vi "serpenbot_DDPG_learing_parallel_old_camera_2.vi"() -> ()   [LabVIEW 2020]
uses:
  <vilib>/Analysis/Matrix/Datatypes/RealMatrix.ctl
  <vilib>/Analysis/Matrix/NI_Matrix.lvlib
  <vilib>/Analysis/NI_AALBase.lvlib
  <vilib>/Analysis/baseanly.llb/Real A x B.vi
  <vilib>/Analysis/NI_AALPro.lvlib
  <vilib>/Analysis/Matrix/Numeric/Subtract/Subtract - RM,RM.vi
  <vilib>/Analysis/_algsub.llb/Real PseudoInverse Matrix.vi
panel:
  out "camera_value 2":T1
  out "appended array 3":T1
  out "error out Y":errorcluster
  out "error out X":errorcluster
  out "laser control value":dbl[](array[numeric])
  out "current y":dbl
  out "current x":dbl
  out "control_loop_time":u32
  in  "stop":bool
  in  "Logging":bool caption="Enable"
  in  "k":T1
  in  "Diode Current\nSetting":dbl=3.0
  in  "Laser Repetition\nFrequency":i32=50000
  in  "VISA resource name":refnum<visa-resource-name>="COM14"
  in  "baud rate (9600)":u32=9600
  out "error out":errorcluster
  out "Identification system 1":string
  out "Conn. axes system 1":string[](array[string])
  out "Identification system 2":string
  out "Conn. axes system  2":string[](array[string])
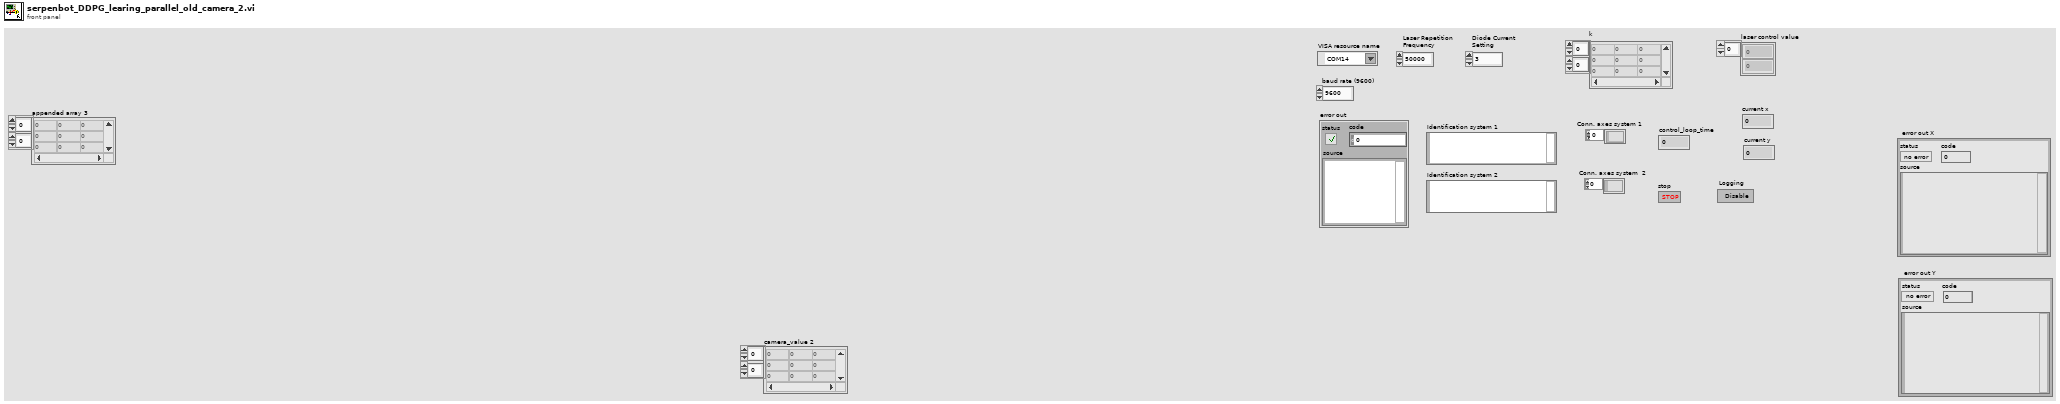
[diagram p1: front panel]
types:
  T1 = typedef "NI_Matrix.lvlib/RealMatrix.ctl" = dbl[][]
  T2 = cluster{"RS232 settings":cluster{"Portnumber":i32, "Baudrate":u16}, "USB settings":cluster{"S/N":string, "USB Search?":bool}, "TCP/IP settings":cluster{"Host address/name":string, "Port":i32, "Board":i32, "TCP/IP Search?":bool}}
  T3 = cluster{"Check FRF?":bool, "Referencing mode":enum16{"FRF (-> FNL)", "FRF", "FNL", "FPL", "RON OFF"}[]}
  T4 = cluster{"Force?":bool, "Dialog?":bool, "Stages":string[]}
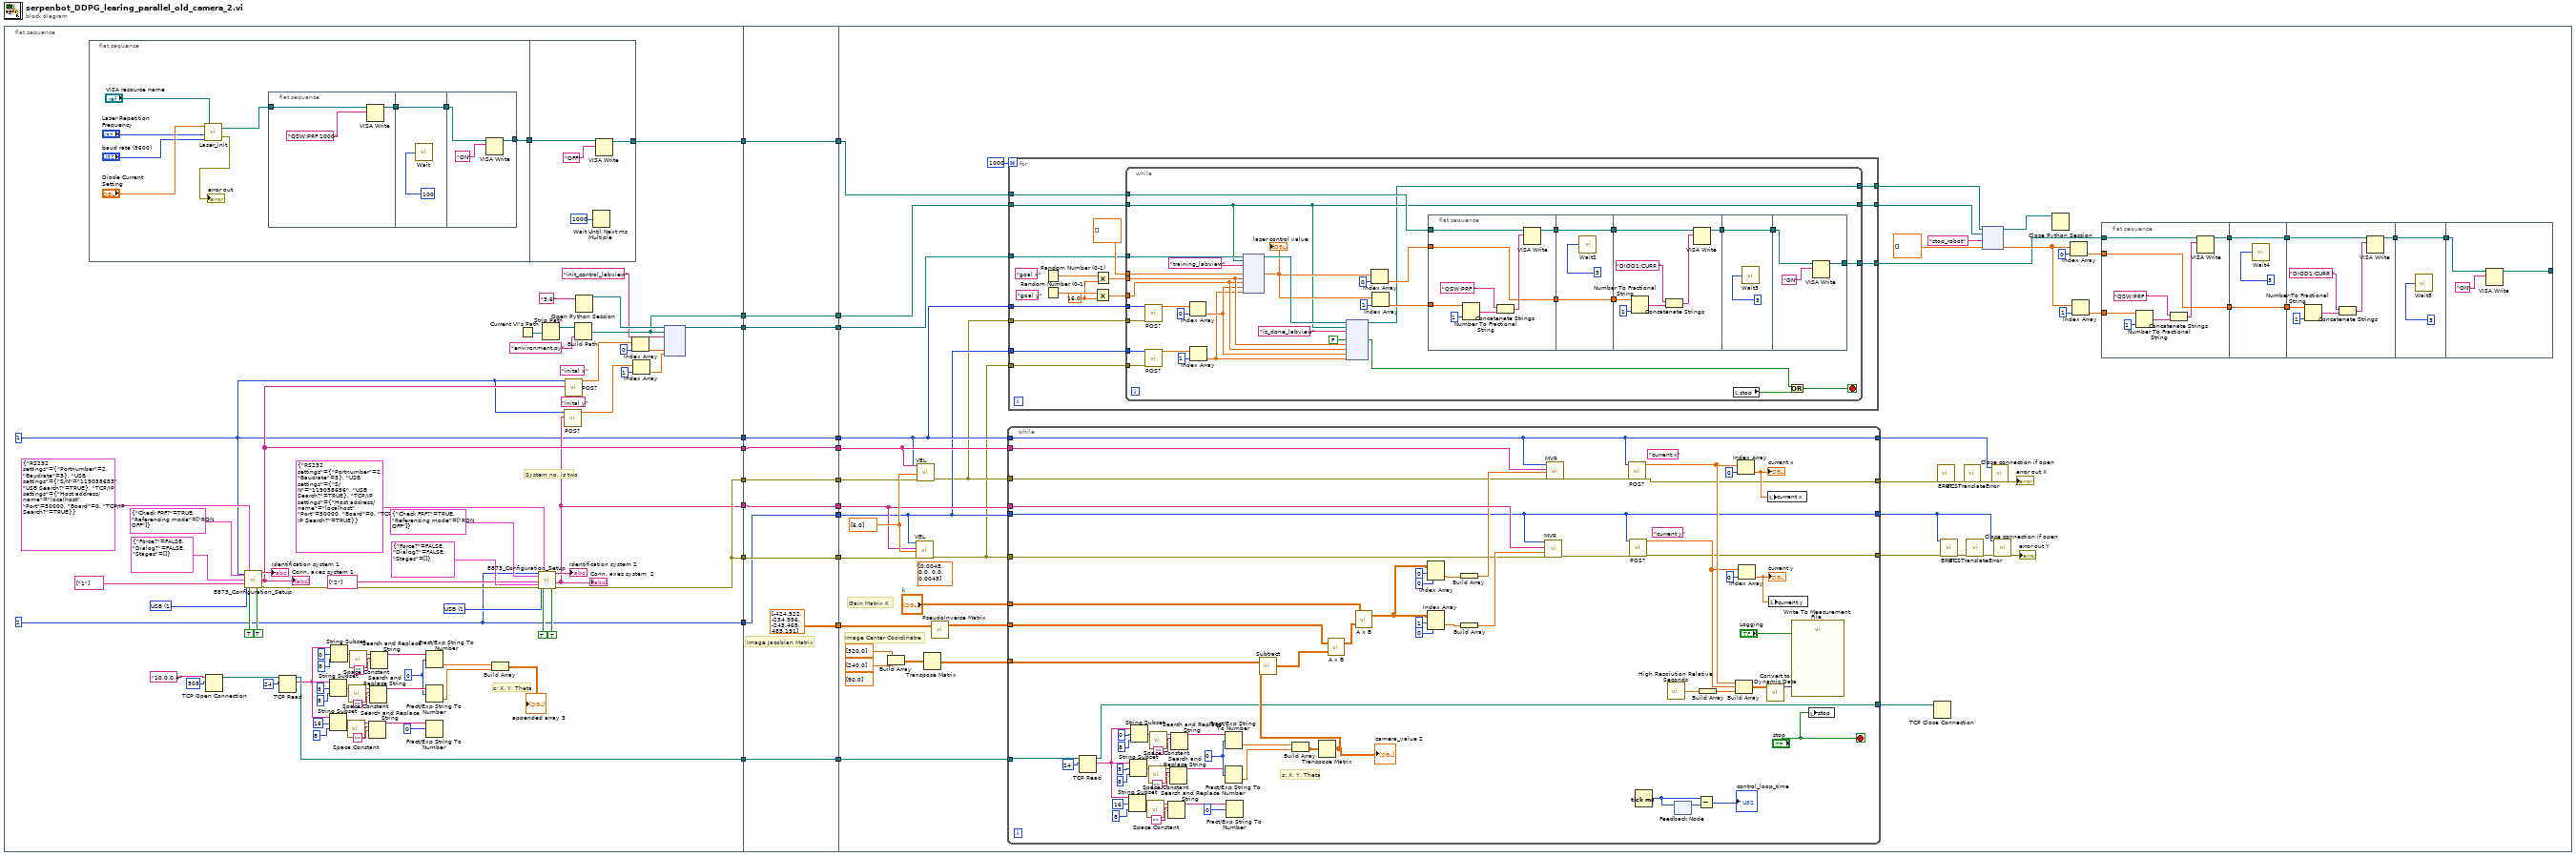
[diagram p0: block diagram]
diagram:
  n1 = flat-sequence {
    tunnel: [w87] -> w21
    tunnel: [w57] -> w20
    tunnel: [w59] -> w19
    tunnel: [w68] -> w18
    tunnel: [w58] -> w17
    tunnel: [w69] -> w16
    tunnel: [w68] -> w15
    tunnel: [w61] -> w14
    tunnel: [w60] -> w13
    tunnel: [w22] -> w2
    tunnel: w21 -> [w120]
    tunnel: [w120] -> w12
    tunnel: w20 -> [w119]
    tunnel: w19 -> [w118]
    tunnel: w18 -> [w117]
    tunnel: w17 -> [w116]
    tunnel: w16 -> [w114]
    tunnel: [w119] -> w11
    tunnel: [w118] -> w10
    tunnel: [w117] -> w9
    tunnel: [w116] -> w8
    tunnel: w15 -> [w115]
    tunnel: [w115] -> w7
    tunnel: [w114] -> w6
    tunnel: [T1 [[-424.522, -234.956], [-243.465, 485.191]] ("J_init 2")] -> w5
    tunnel: w14 -> [w112]
    tunnel: w13 -> [w111]
    tunnel: [w112] -> w4
    tunnel: [w111] -> w3
    tunnel: w2 -> [w110]
    tunnel: [w110] -> w1
    tunnel: w12 -> [w141]
    tunnel: w11 -> [w125]
    tunnel: w10 -> [w162]
    tunnel: w9 -> [w165]
    tunnel: w8 -> [w161]
    tunnel: w7 -> [w164]
    tunnel: w6 -> [w124]
    tunnel: w5 -> [w163]
    tunnel: w4 -> [w143]
    tunnel: w3 -> [w142]
    tunnel: w1 -> [w127]
    frame #0 {
      w36 = 0
      (unwired) "inital y"
      (unwired) "inital x"
      w72 = u16 1 items=["RS232", "USB", "TCP/IP"] ("Interface")
      w75 = u16 1 items=["RS232", "USB", "TCP/IP"] ("Interface")
      w69 = 2 ("System no.")
      w57 = 1 ("System no.")
      # "s: X, Y, Theta"
      # "System no. is two"
      n2 = flat-sequence {
        tunnel: [w89] -> w88
        tunnel: w88 -> [w107]
        tunnel: [w106] -> w87
        frame #0 {
          n3 = call "Laser_init.vi"("baud rate (9600)"="baud rate (9600)", "Laser Repetition\nFrequency"="Laser Repetition\nFrequency", "VISA resource name"="VISA resource name", "Diode Current\nSetting"="Diode Current\nSetting") -> ("error out"=→"error out":errorcluster, "VISA Refnum out"=w90:refnum<visa-resource-name>)
          n4 = flat-sequence {
            tunnel: w90 -> [w100]
            tunnel: [w99] -> w97
            tunnel: w97 -> [w102]
            tunnel: [w102] -> w96
            tunnel: w96 -> [w103]
            tunnel: [w104] -> w89
            frame #0 {
              n5 = VISA Write(VISA resource name=w100, write buffer="QSW:PRF 1000" ("string")) -> (VISA resource name out=w99:refnum<visa-resource-name>)  [unwired: 1 in, 2 out]
            }
            frame #1 {
              n6 = call "Wait"("Count(mSec)"=u32 100) -> ()  [unwired: 1 out]
            }
            frame #2 {
              n7 = VISA Write(VISA resource name=w103, write buffer="ON") -> (VISA resource name out=w104:refnum<visa-resource-name>)  [unwired: 1 in, 2 out]
            }
          }
        }
        frame #1 {
          n8 = Wait Until Next ms Multiple(millisecond multiple=u32 1000) -> ()  [unwired: 1 out]
          n9 = VISA Write(VISA resource name=w107, write buffer="OFF") -> (VISA resource name out=w106:refnum<visa-resource-name>)  [unwired: 1 in, 2 out]
        }
      }
      n10 = TCP Open Connection(address="10.0.0.4", remote port or service name=u16 503) -> (connection ID=w46:refnum<k5>)  [unwired: 3 in, 1 out]
      n11 = call "E873_Configuration_Setup.vi"("System no."=w57, "Referencing"=T3 {"Check FRF?"=TRUE, "Referencing mode"=[enum."RON OFF"]}, "Interface"=w75, "All axes?"=TRUE, "Axes to move"=string[] ["1"], "Interface settings"=T2 {"RS232 settings"={"Portnumber"=2, "Baudrate"=5}, "USB settings"={"S/N"="119058653", "USB Search?"=TRUE}, "TCP/IP settings"={"Host address/name"="localhost", "Port"=50000, "Board"=0, "TCP/IP Search?"=TRUE}}, "Stage selection"=T4 {"Force?"=FALSE, "Dialog?"=FALSE, "Stages"=[]}, "Switch servo on?"=TRUE ("Use dialog to define\nconnected stages?")) -> ("Identification"=→"Identification system 1":string, "Conn. \nAxes"=w59:string[], "error out"=w84:errorcluster)  [unwired: 4 in, 5 out]
      "Conn. axes system 1" <- w59
      n12 = TCP Read(connection ID=w46, bytes to read=24) -> (connection ID out=w22:refnum<k5>, data out=w45:string)  [unwired: 3 in, 1 out]
      n13 = String Subset(string=w45, offset (0)=16, length (rest)=8 ("length (rest)")) -> (substring=w43:string)
      n14 = String Subset(string=w45, offset (0)=8, length (rest)=8 ("length (rest)")) -> (substring=w44:string)
      n15 = String Subset(string=w45, offset (0)=0, length (rest)=8 ("length (rest)")) -> (substring=w42:string)
      n16 = call <vilib>:"Space Constant.vi"() -> ("String"=w41:string)
      n17 = call <vilib>:"Space Constant.vi"() -> ("String"=w40:string)
      n18 = call <vilib>:"Space Constant.vi"() -> ("String"=w39:string)
      n19 = Search and Replace String(input string=w43, search string=w41, replace string="") -> (result string=w47:string)  [unwired: 5 in, 3 out]
      n20 = Search and Replace String(input string=w44, search string=w40, replace string="") -> (result string=w48:string)  [unwired: 5 in, 3 out]
      n21 = Search and Replace String(input string=w42, search string=w39, replace string="") -> (result string=w49:string)  [unwired: 5 in, 3 out]
      n22 = Fract/Exp String To Number(string=w49, offset=w36) -> (number=w37:dbl)  [unwired: 2 in, 1 out]
      n23 = Fract/Exp String To Number(string=w48, offset=w36) -> (number=w38:dbl)  [unwired: 2 in, 1 out]
      n24 = Fract/Exp String To Number(string=w47, offset=0) -> ()  [unwired: 2 in, 2 out]
      n25 = Build Array(w37, w38) -> (→"appended array 3":T1)
      n26 = Current VI's Path() -> (path=w67:path)
      n27 = call "E873_Configuration_Setup.vi"("System no."=w69, "Referencing"=T3 {"Check FRF?"=TRUE, "Referencing mode"=[enum."RON OFF"]}, "Interface"=w72, "All axes?"=TRUE, "Axes to move"=string[] ["2"], "error in"=w84, "Interface settings"=T2 {"RS232 settings"={"Portnumber"=2, "Baudrate"=5}, "USB settings"={"S/N"="119058656", "USB Search?"=TRUE}, "TCP/IP settings"={"Host address/name"="localhost", "Port"=50000, "Board"=0, "TCP/IP Search?"=TRUE}}, "Stage selection"=T4 {"Force?"=FALSE, "Dialog?"=FALSE, "Stages"=[]}, "Switch servo on?"=TRUE ("Use dialog to define\nconnected stages?")) -> ("Identification"=→"Identification system 2":string, "Conn. \nAxes"=w58:string[], "error out"=w68:errorcluster)  [unwired: 3 in, 5 out]
      "Conn. axes system  2" <- w58
      n28 = Strip Path(path=w67) -> (stripped path=w66:path)  [unwired: 1 out]
      n29 = call "POS?.vi"("System no."=w57, "Axes to query"=w58) -> ("Position"=w51:dbl[])  [unwired: 3 in, 14 out]
      n30 = call "POS?.vi"("System no."=w57, "Axes to query"=w59) -> ("Position"=w54:dbl[])  [unwired: 3 in, 14 out]
      n31 = Build Path(base path=w66, name or relative path="environment.py") -> (appended path=w61:path)
      n32 = Open Python Session(python version="3.6" ("Python version")) -> (session out=w63:refnum<k35>)  [unwired: 2 in, 1 out]
      n33 = Index Array(array=w54, index=0) -> (element=w55:dbl)
      n34 = Index Array(array=w51, index=1) -> (element=w52:dbl)
      n35 = node(w63, w61, "init_control_labview" ("function name"), w55, w52) -> (w60:refnum<k35>)  [unwired: 5 in, 3 out]
    }
    frame #1 {
      # "Image Jacobian Matrix"
    }
    frame #2 {
      w166 = dbl[] [6.0] ("Velocity values")
      (unwired) T1 [[0.0045, 0.0], [0.0, 0.0045]] ("J_init 2")
      (unwired) dbl[] [90.0] ("element")
      # "Gain Matrix K"
      # "Image Center Coordinatre"
      n36 = Build Array(dbl[] [320.0] ("element"), dbl[] [240.0] ("element")) -> (w167:T1)
      n37 = call "VEL.vi"("System no."=w124, "Axes to set"=w161, "Velocity values"=w166, "error in"=w164) -> ("error out"=w122:errorcluster)  [unwired: 2 in, 13 out]
      n38 = call "VEL.vi"("System no."=w125, "Axes to set"=w162, "Velocity values"=w166, "error in"=w165) -> ("error out"=w123:errorcluster)  [unwired: 2 in, 13 out]
      n39 = Transpose Matrix(1:w167) -> (0:w158:T1)
      n40 = call-poly <vilib>:"PseudoInverse Matrix.vi"("Input Matrix"=w163) -> ("PseudoInverse Matrix"=w159:T1)  [unwired: 1 in, 1 out]
      n41 = while {
        tunnel: w122 -> [w293]
        tunnel: w124 -> [w274]
        tunnel: w161 -> [w311]
        tunnel: w123 -> [w294]
        tunnel: w162 -> [w310]
        tunnel: w125 -> [w276]
        tunnel: w159 -> [w299]
        tunnel: "k" -> [w298]
        tunnel: w158 -> [w297]
        tunnel: [w276] -> w130
        tunnel: [w275] -> w121
        tunnel: [w274] -> w129
        tunnel: [w273] -> w128
        tunnel: w127 -> [w246]
        tunnel: [w245] -> w126
        stop <- "stop" stop-if-true
        w272 = 0
        (unwired) "current y"
        (unwired) "current x"
        # "s: X, Y, Theta"
        n42 = TCP Read(connection ID=w246, bytes to read=24) -> (connection ID out=w245:refnum<k5>, data out=w253:string)  [unwired: 3 in, 1 out]
        n43 = String Subset(string=w253, offset (0)=16, length (rest)=8 ("length (rest)")) -> (substring=w255:string)
        n44 = String Subset(string=w253, offset (0)=8, length (rest)=8 ("length (rest)")) -> (substring=w254:string)
        n45 = String Subset(string=w253, offset (0)=0, length (rest)=8 ("length (rest)")) -> (substring=w260:string)
        n46 = call <vilib>:"Space Constant.vi"() -> ("String"=w263:string)
        n47 = call <vilib>:"Space Constant.vi"() -> ("String"=w265:string)
        n48 = call <vilib>:"Space Constant.vi"() -> ("String"=w267:string)
        n49 = Search and Replace String(input string=w255, search string=w263, replace string="") -> (result string=w251:string)  [unwired: 5 in, 3 out]
        n50 = Search and Replace String(input string=w254, search string=w265, replace string="") -> (result string=w250:string)  [unwired: 5 in, 3 out]
        n51 = Search and Replace String(input string=w260, search string=w267, replace string="") -> (result string=w249:string)  [unwired: 5 in, 3 out]
        n52 = Fract/Exp String To Number(string=w249, offset=w272) -> (number=w271:dbl)  [unwired: 2 in, 1 out]
        n53 = Fract/Exp String To Number(string=w250, offset=w272) -> (number=w270:dbl)  [unwired: 2 in, 1 out]
        n54 = Fract/Exp String To Number(string=w251, offset=0) -> ()  [unwired: 2 in, 2 out]
        n55 = Build Array(w271, w270) -> (w248:T1)
        n56 = Transpose Matrix(1:w248) -> (0:w247:T1)
        "camera_value 2" <- w247
        n57 = call-poly <vilib>:"Subtract.vi"("Real Matrix B"=w247, "Real Matrix A"=w297) -> ("A - B"=w305:T1)
        n58 = call-poly <vilib>:"A x B.vi"("B"=w305, "A"=w299) -> ("A x B"=w303:T1)  [unwired: 1 out]
        n59 = call-poly <vilib>:"A x B.vi"("B"=w303, "A"=w298) -> ("A x B"=w304:T1)  [unwired: 1 out]
        n60 = Index Array(array=w304, index (row)=0, index (col)=0) -> (element=w296:dbl)
        n61 = Index Array(array=w304, index (row)=1, index (col)=0) -> (element=w295:dbl)
        n62 = Build Array(w296) -> (w302:dbl[])
        n63 = Build Array(w295) -> (w301:dbl[])
        n64 = call "MVR.vi"("System no."=w274, "Axes to move"=w311, "Position values"=w301, "error in"=w293) -> ("error out"=w285:errorcluster)  [unwired: 1 in, 14 out]
        n65 = call "MVR.vi"("System no."=w276, "Axes to move"=w310, "Position values"=w302, "error in"=w294) -> ("error out"=w286:errorcluster)  [unwired: 1 in, 14 out]
        n66 = call "POS?.vi"("System no."=w276, "error in"=w286) -> ("Position"=w283:dbl[], "error out"=w275:errorcluster)  [unwired: 3 in, 13 out]
        n67 = call "POS?.vi"("System no."=w274, "error in"=w285) -> ("Position"=w281:dbl[], "error out"=w273:errorcluster)  [unwired: 3 in, 13 out]
        n68 = Tick Count (ms)() -> (millisecond timer value=w284:u32)
        n69 = call <vilib>:"High Resolution Relative Seconds.vi"() -> ("relative seconds"=w288:dbl)
        n70 = feedback #1() -> (w300:u32)  [unwired: 1 in]
        n71 = feedback-in #1(w284) -> ()
        n72 = Subtract(x=w284, y=w300) -> (x-y=→"control_loop_time":u32)
        n73 = Build Array(w288) -> (w287:dbl[])
        n74 = Build Array(w283, w281, w287) -> (w290:dbl[][])
        n75 = Index Array(array=w283, index=0) -> (element=w279:dbl)
        "current x" <- w279
        n76 = Index Array(array=w281, index=0) -> (element=w278:dbl)
        "current y" <- w278
        n77 = call "Convert to Dynamic Data"("2D Array"=w290) -> ("Dynamic Data Type"=w289:dynamicdata)  [unwired: 3 in]
        n78 = local write "current x"(w279) -> ()
        n79 = local write "current y"(w278) -> ()
        n80 = call "Write To Measurement File"("Signals"=w289, "Enable"="Logging") -> ()  [unwired: 15 in, 3 out]
        n81 = local write "stop"("stop") -> ()
      }
      n82 = for {
        N: 1000 -> [_]
        tunnel: w143 -> [w179]
        tunnel: w142 -> [w178]
        tunnel: w141 -> [w177]
        tunnel: [w176] -> w139
        tunnel: [w175] -> w138
        tunnel: [w174] -> w137
        tunnel: w125 -> [w173]
        tunnel: w124 -> [w172]
        tunnel: w123 -> [w171]
        tunnel: w122 -> [w170]
        w183 = 16.0
        (unwired) "goal y"
        (unwired) "goal x"
        n83 = Random Number (0-1)() -> (number: 0 to 1=w185:dbl)
        n84 = Random Number (0-1)() -> (number: 0 to 1=w184:dbl)
        n85 = Multiply(x=w184, y=w183) -> (x*y=w180:dbl)
        n86 = Multiply(x=w185, y=w183) -> (x*y=w181:dbl)
        n87 = while {
          tunnel: dbl[] [] -> [w206]
          tunnel: w181 -> [w205]
          tunnel: w180 -> [w204]
          tunnel: w179 -> [w201]
          tunnel: w178 -> [w203]
          tunnel: w177 -> [w202]
          tunnel: [w201] -> w176
          tunnel: [w200] -> w175
          tunnel: [w197] -> w174
          tunnel: w173 -> [w192]
          tunnel: w172 -> [w188]
          tunnel: w171 -> [w187]
          tunnel: w170 -> [w186]
          stop <- w198 stop-if-true
          n88 = call "POS?.vi"("System no."=w192, "error in"=w187) -> ("Position"=w194:dbl[])  [unwired: 3 in, 14 out]
          n89 = call "POS?.vi"("System no."=w188, "error in"=w186) -> ("Position"=w190:dbl[])  [unwired: 3 in, 14 out]
          n90 = Index Array(array=w194, index=0) -> (element=w193:dbl)
          n91 = Index Array(array=w190, index=1) -> (element=w189:dbl)
          n92 = node(w203, w201, "training_labview" ("function name"), w206, w205, w204, w193, w189) -> (w214:refnum<k35>, w208:dbl[])  [unwired: 5 in, 3 out]
          "laser control value" <- w208
          n93 = node(w214, w201, "is_done_labview" ("function name"), FALSE, w205, w204, w193, w189) -> (w200:refnum<k35>, w196:bool)  [unwired: 5 in, 3 out]
          n94 = Index Array(array=w208, index=0) -> (element=w211:dbl)
          n95 = Index Array(array=w208, index=1) -> (element=w207:dbl)
          n96 = flat-sequence {
            tunnel: w202 -> [w225]
            tunnel: [w224] -> w221
            tunnel: w207 -> [w223]
            tunnel: w211 -> [w222]
            tunnel: [w222] -> w220
            tunnel: [w232] -> w219
            tunnel: [w230] -> w218
            tunnel: w221 -> [w232]
            tunnel: w220 -> [w230]
            tunnel: [w239] -> w217
            tunnel: w219 -> [w237]
            tunnel: w218 -> [w234]
            tunnel: w217 -> [w241]
            tunnel: [w241] -> w216
            tunnel: w216 -> [w243]
            tunnel: [w242] -> w197
            frame #0 {
              n97 = Number To Fractional String(number=w223, precision (6)=i16 1) -> (F-format string=w228:string)  [unwired: 2 in]
              n98 = Concatenate Strings("QSW:PRF " ("string"), w228) -> (w229:string)
              n99 = VISA Write(VISA resource name=w225, write buffer=w229) -> (VISA resource name out=w224:refnum<visa-resource-name>)  [unwired: 1 in, 2 out]
            }
            frame #1 {
              n100 = call "Wait2"("Count(mSec)"=u32 3) -> ()  [unwired: 1 out]
            }
            frame #2 {
              n101 = Number To Fractional String(number=w234, precision (6)=i16 1) -> (F-format string=w235:string)  [unwired: 2 in]
              n102 = Concatenate Strings("DIOD1:CURR " ("string"), w235) -> (w238:string)
              n103 = VISA Write(VISA resource name=w237, write buffer=w238) -> (VISA resource name out=w239:refnum<visa-resource-name>)  [unwired: 1 in, 2 out]
            }
            frame #3 {
              n104 = call "Wait3"("Count(mSec)"=u32 3) -> ()  [unwired: 1 out]
            }
            frame #4 {
              n105 = VISA Write(VISA resource name=w243, write buffer="ON") -> (VISA resource name out=w242:refnum<visa-resource-name>)  [unwired: 1 in, 2 out]
            }
          }
          n106 = local read "stop"() -> (w199:bool)
          n107 = Or(x=w196, y=w199) -> (x .or. y?=w198:bool)
        }
      }
      n108 = TCP Close Connection(connection ID=w126) -> ()  [unwired: 2 in, 2 out]
      n109 = call "ERR?.vi"("error in"=w121) -> ("error out"=w134:errorcluster)  [unwired: 1 in, 17 out]
      n110 = call "ERR?.vi"("System no."=w129, "error in"=w128) -> ("error out"=w131:errorcluster)  [unwired: 17 out]
      n111 = call "GCSTranslateError.vi"("error in"=w134) -> ("error out"=w135:errorcluster)  [unwired: 18 out]
      n112 = call "GCSTranslateError.vi"("error in"=w131) -> ("error out"=w132:errorcluster)  [unwired: 18 out]
      n113 = node(w138, w139, "stop_robot" ("function name"), dbl[] []) -> (w149:refnum<k35>, w144:dbl[])  [unwired: 1 in, 3 out]
      n114 = call "Close connection if open.vi"("System no."=w130, "error in"=w135) -> ("error out"=→"error out X":errorcluster)  [unwired: 1 in, 16 out]
      n115 = call "Close connection if open.vi"("System no."=w129, "error in"=w132) -> ("error out"=→"error out Y":errorcluster)  [unwired: 1 in, 16 out]
      n116 = Close Python Session(session in=w149) -> ()  [unwired: 1 in, 1 out]
      n117 = Index Array(array=w144, index=0) -> (element=w146:dbl)
      n118 = Index Array(array=w144, index=1) -> (element=w145:dbl)
      n119 = flat-sequence {
        tunnel: w137 -> [w315]
        tunnel: [w314] -> w157
        tunnel: w145 -> [w313]
        tunnel: w146 -> [w312]
        tunnel: [w312] -> w156
        tunnel: [w322] -> w155
        tunnel: [w320] -> w154
        tunnel: w157 -> [w322]
        tunnel: w156 -> [w320]
        tunnel: [w329] -> w153
        tunnel: w155 -> [w327]
        tunnel: w154 -> [w324]
        tunnel: w153 -> [w331]
        tunnel: [w331] -> w152
        tunnel: w152 -> [w333]
        tunnel: [w332] -> _
        frame #0 {
          n120 = Number To Fractional String(number=w313, precision (6)=i16 1) -> (F-format string=w318:string)  [unwired: 2 in]
          n121 = Concatenate Strings("QSW:PRF " ("string"), w318) -> (w319:string)
          n122 = VISA Write(VISA resource name=w315, write buffer=w319) -> (VISA resource name out=w314:refnum<visa-resource-name>)  [unwired: 1 in, 2 out]
        }
        frame #1 {
          n123 = call "Wait4"("Count(mSec)"=u32 3) -> ()  [unwired: 1 out]
        }
        frame #2 {
          n124 = Number To Fractional String(number=w324, precision (6)=i16 1) -> (F-format string=w325:string)  [unwired: 2 in]
          n125 = Concatenate Strings("DIOD1:CURR " ("string"), w325) -> (w328:string)
          n126 = VISA Write(VISA resource name=w327, write buffer=w328) -> (VISA resource name out=w329:refnum<visa-resource-name>)  [unwired: 1 in, 2 out]
        }
        frame #3 {
          n127 = call "Wait5"("Count(mSec)"=u32 3) -> ()  [unwired: 1 out]
        }
        frame #4 {
          n128 = VISA Write(VISA resource name=w333, write buffer="ON") -> (VISA resource name out=w332:refnum<visa-resource-name>)  [unwired: 1 in, 2 out]
        }
      }
    }
  }
